vi "PathPlanner_PointTowardsZone_FromJSON.vi"(11 "JSON String":string) -> (1 "Exists":bool, 3 "PointTowardsZones":T2[](array[typedef]) {"TargetPosition"."Y" format="%14.3f"; "TargetPosition"."X" format="%14.3f"; "RotationOffset"."SIN" format="%13.4f"; "RotationOffset"."COS" format="%13.4f"; "RotationOffset"."VALUE" format="%13.4f"})   [LabVIEW 2019, in "PathPlanner24.lvlib"]
doc: "Create a constraints zone from json\n \nInputs: \n -- JsonString - string - String containing the JSON to parse.\n\nOutputs:\n -- ConstraintsZone - cluster - The constraints zone defined by the given json object\n -- Exists -- boolean -- True if a constraints zone was found and parsed."
uses:
  PathPlanner24.lvlib
  <vilib>/Rock Robotics/WPI/ThirdParty/JAS_Junk/TrajLib/Trajectory_Library.lvlib
  <vilib>/Rock Robotics/WPI/ThirdParty/JAS_Junk/TrajLib/TypeDef/TRANSLATION2D.ctl
  <vilib>/Rock Robotics/WPI/ThirdParty/JAS_Junk/TrajLib/TypeDef/ROTATION2D.ctl
  TypeDef/PathPlannerPointTowardsZone.ctl
panel:
  in  "pointTowardsZones":T1(array[cluster])
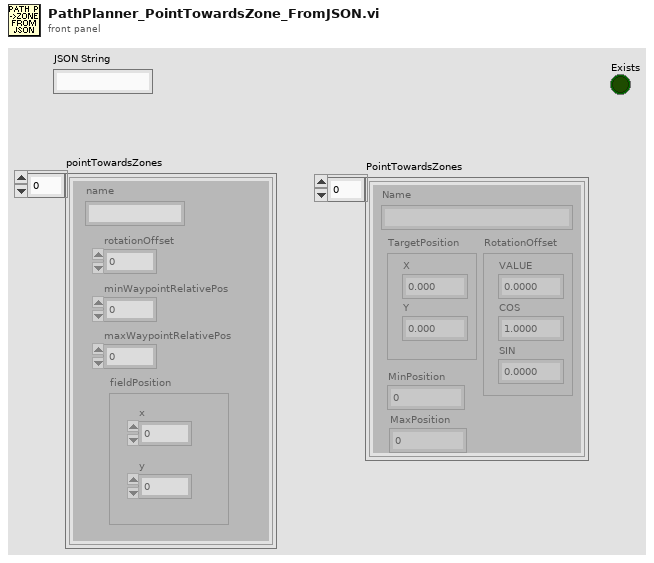
[diagram p1: front panel]
types:
  T1 = cluster{"name":string, "rotationOffset":dbl, "minWaypointRelativePos":dbl, "fieldPosition":cluster{"x":dbl, "y":dbl}, "maxWaypointRelativePos":dbl}[]
  T2 = typedef "PathPlanner24.lvlib/PathPlannerPointTowardsZone.ctl" = cluster{"RotationOffset":T3, "Name":string, "TargetPosition":T4, "MinPosition":dbl, "MaxPosition":dbl}
  T3 = typedef "Trajectory_Library.lvlib/ROTATION2D.ctl" = cluster{"VALUE":dbl, "COS":dbl, "SIN":dbl}
  T4 = typedef "Trajectory_Library.lvlib/TRANSLATION2D.ctl" = cluster{"X":dbl, "Y":dbl}
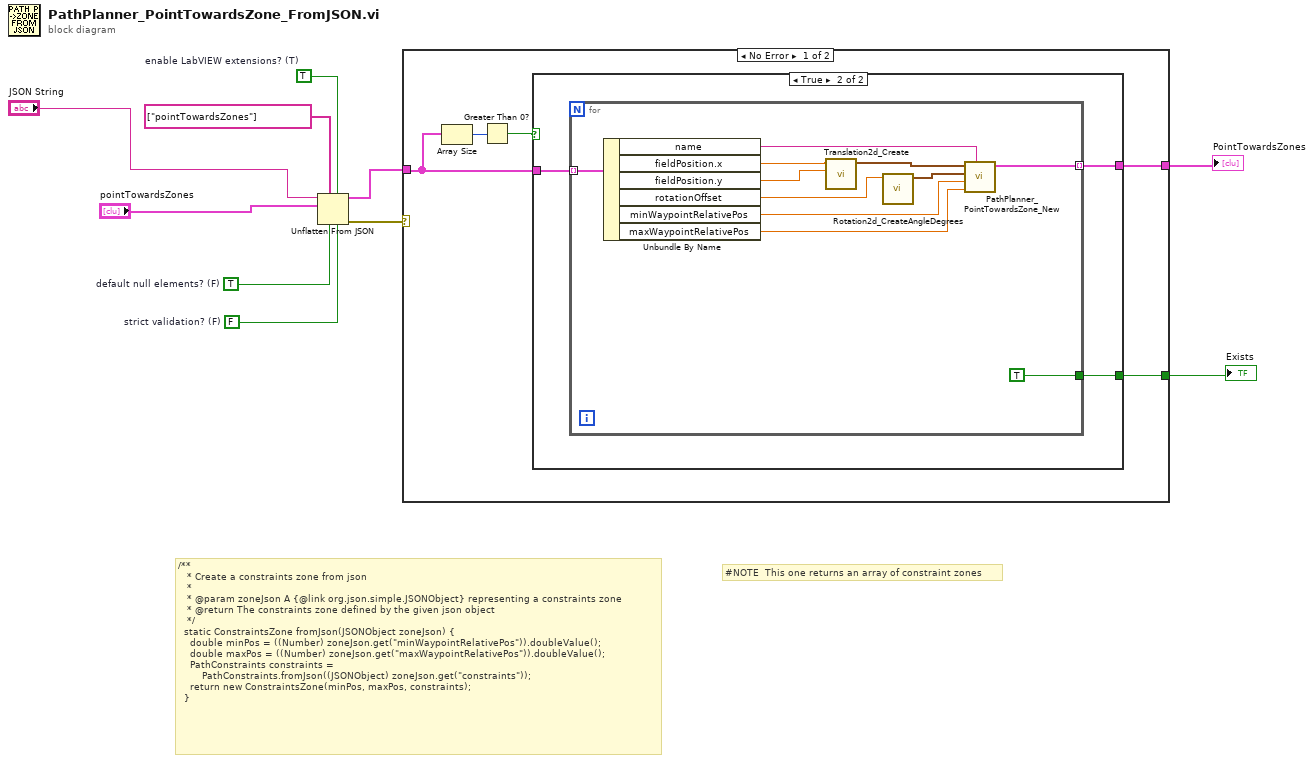
[diagram p0: block diagram]
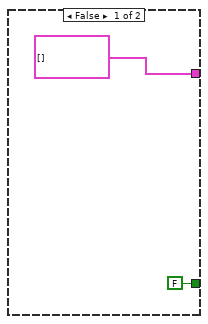
[diagram p2: hidden frame]
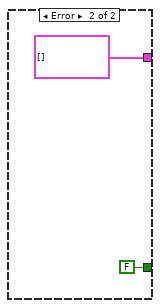
[diagram p3: hidden frame]
diagram:
  w5 = FALSE  # strict validation? (F)
  w6 = TRUE  # default null elements? (F)
  w7 = TRUE  # enable LabVIEW extensions? (T)
  # "#NOTE  This one returns an array of constraint zones"
  # "/**\n   * Create a constraints zone from json\n   *\n   * @param zoneJson A {@link org.json.simple.JSONObject} representing a constraints zone\n   * @return The constraints zone defined by the given json object\n   */\n  static ConstraintsZone fromJson(JSONObject zoneJson) {\n    double minPos = ((Number) zoneJson.get(\"minWaypointRelativePos\")).doubleValue();\n    double maxPos = ((Number) zoneJson.get(\"maxWaypointRelativePos\")).doubleValue();\n    PathConstraints constraints =\n        PathConstraints.fromJson((JSONObject) zoneJson.get(\"constraints\"));\n    return new ConstraintsZone(minPos, maxPos, constraints);\n  }"
  n1 = Unflatten From JSON(path=string[] ["pointTowardsZones"] ("path 5"), enable LabVIEW extensions? (T)=w7, JSON string="JSON String", type and defaults="pointTowardsZones", default null elements? (F)=w6, strict validation? (F)=w5) -> (value=w3:T1, error out=w4:errorcluster)  [unwired: 1 in]
  n2 = case shown="No Error" w4 {
    tunnel: w3 -> [w13 _]
    tunnel: [w12 FALSE] -> w2
    tunnel: [w11 T2[] [] ("PointTowardsZones")] -> w1
    frame No Error {
      n3 = Array Size(array=w13) -> (size(s)=w15:i32)
      n4 = Greater Than 0?(x=w15) -> (x > 0?=w14:bool)
      n5 = case shown="True" w14 {
        tunnel: w13 -> [_ w20]
        tunnel: [T2[] [] ("PointTowardsZones") w18] -> w11
        tunnel: [FALSE w19] -> w12
        frame False {
        }
        frame True {
          n6 = for {
            tunnel: w20 -> [w31] mode=indexing
            tunnel: [TRUE] -> w19
            tunnel: [w21] -> w18 mode=indexing
            n7 = Unbundle By Name(w31) -> ("name"=w29:string, "fieldPosition.x"=w28:dbl, "fieldPosition.y"=w27:dbl, "rotationOffset"=w25:dbl, "minWaypointRelativePos"=w23:dbl, "maxWaypointRelativePos"=w22:dbl)
            n8 = call <vilib>:"Translation2d_Create.vi"("Y"=w27, "X"=w28) -> ("TRANSLATION"=w26:T4)  [unwired: 9 in]
            n9 = call <vilib>:"Rotation2d_CreateAngleDegrees.vi"("Angle_Degrees"=w25) -> ("ROTATION"=w24:T3)  [unwired: 10 in]
            n10 = call "PathPlanner_PointTowardsZone_New.vi"("Name"=w29, "MaxPosition"=w22, "MinPosition"=w23, "RotationOffset"=w24, "TargetPosition"=w26) -> ("PointTowardsZone"=w21:T2)  [unwired: 6 in]
          }
        }
      }
    }
    frame Error {
    }
  }
  "PointTowardsZones" <- w1
  "Exists" <- w2
